vi "Untitled 3.vi"() -> ()   [LabVIEW 2009]
panel:
  in  "Array 2":dbl[][](array[numeric])
  in  "w":dbl
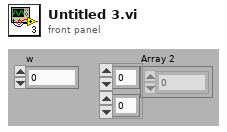
[diagram p1: front panel]
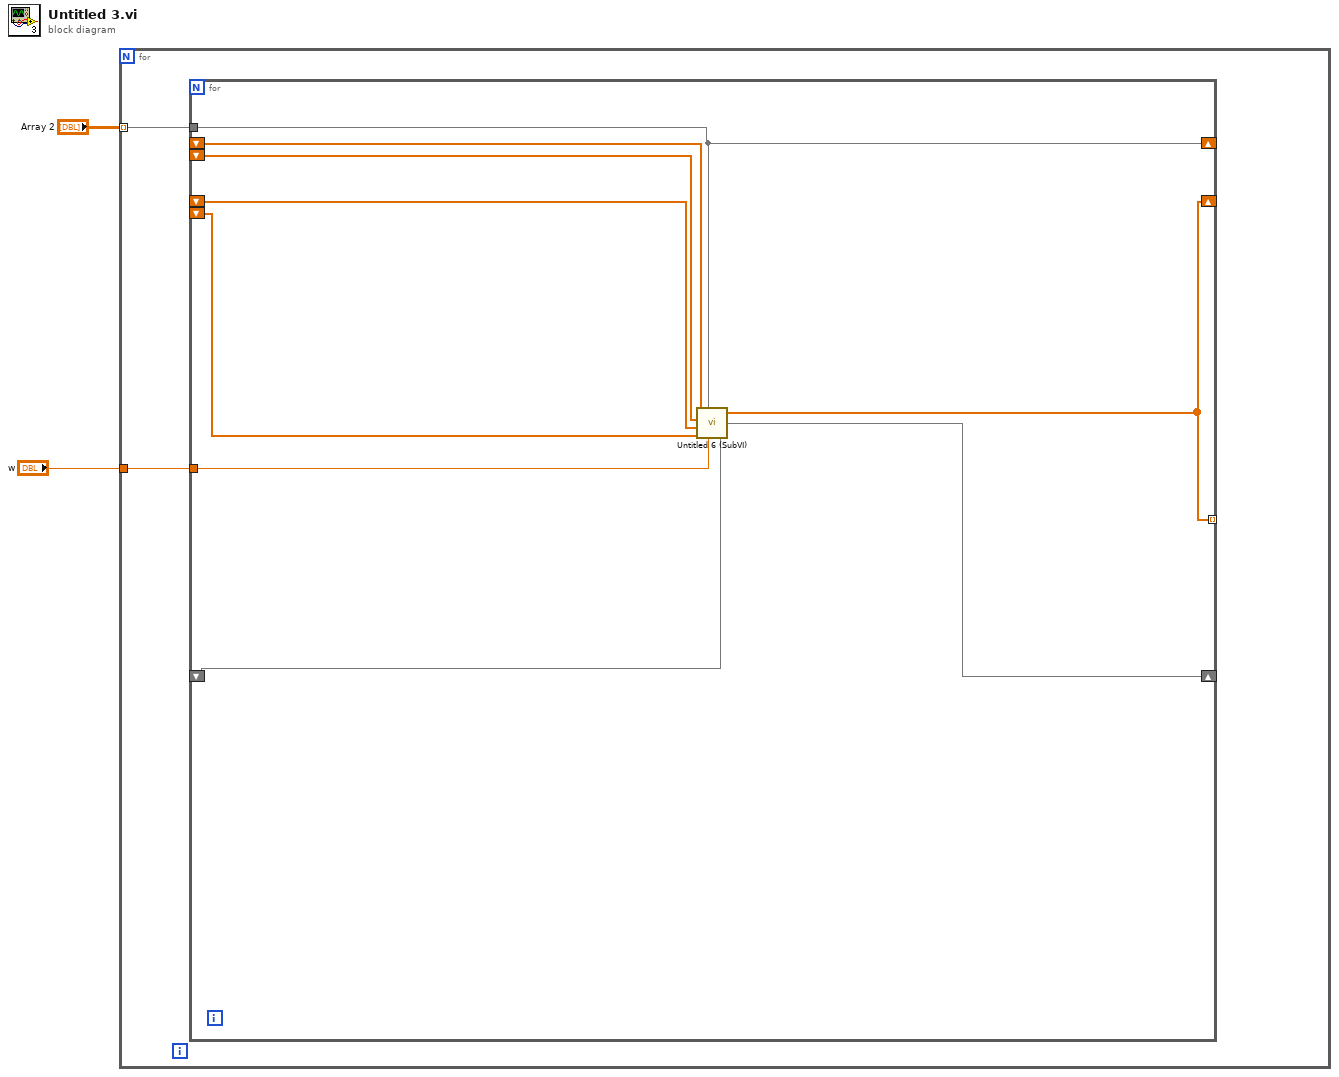
[diagram p0: block diagram]
diagram:
  n1 = for {
    tunnel: "Array 2" -> [w4] mode=indexing
    tunnel: "w" -> [w3]
    n2 = for {
      tunnel: w4 -> [w5]
      shift-right: [w5] -> _
      shift-left: _ -> [w12]
      shift-left: _ -> [w11]
      shift-right: [w13] -> _
      shift-left: _ -> [w10]
      shift-left: _ -> [w9]
      tunnel: [w13] -> _ mode=indexing
      tunnel: w3 -> [w8]
      shift-right: [w7] -> _
      shift-left: _ -> [w6]
      n3 = call "Untitled 6 (SubVI).vi"("x(t-1)"=w12, "x(t)"=w5, "x(t-2)"=w11, "y(t-1)"=w10, "smooth window size"=w8, "y(t-2)"=w9, "RC y(t-1)"=w6) -> ("smoothed data"=w13:dbl[], 7:w7)
    }
  }
